vi "fpga_setup_and_start.vi"(8 "error in":errorcluster, 10 "Bit rate":dbl=400000.0 min=40000.0 max=2000000.0 format="%#_3p") -> (0 "error out":errorcluster, 2 "I2C interface":T1)   [LabVIEW 2013]
uses:
  i2c_interface.ctl
  fpga_reference.ctl
panel:
  # "Open I2C FPGA interface, starting hardware."
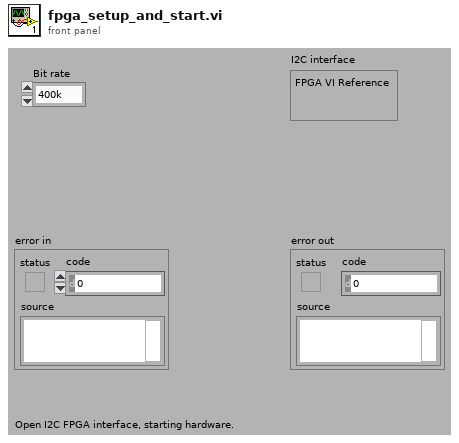
[diagram p1: front panel]
types:
  T1 = typedef "i2c_interface.ctl" = cluster{"FPGA VI Reference":T2}
  T2 = typedef "fpga_reference.ctl" = refnum<k20>
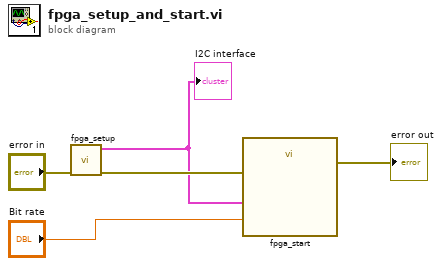
[diagram p0: block diagram]
diagram:
  n1 = call "fpga_setup.vi"("error in"="error in") -> ("error out"=w5:errorcluster, "Cluster"=w1:cluster{"FPGA VI Reference Out":T2})  [unwired: 9 in]
  "I2C interface" <- w1
  n2 = call "fpga_start.vi"("error in"=w5, "Bit rate"="Bit rate", "I2C interface"=w1) -> ("error out"=→"error out":errorcluster)  [unwired: 8 in]
